vi "constants3.vi"() -> ()   [LabVIEW 2020]
panel:
  out "Robot_Width (in)":dbl
  out "Robot_Length (in)":dbl
  out "Angle_from_LL_to_Horizontal (deg)":dbl
  out "Height_from_LL_To_Ground_(in)":dbl
  out "Legal_Shooter_Setpoints":string[](array[string])
  out "Legal_Pipelines":string[](array[string])
  out "Legal_Actuator_Names":string[](array[string])
  out "Legal_Drivers":string[](array[string])
  out "Legal_Robots":string[](array[string])
  out "Legal_Auto_Plays":string[](array[string])
  out "Max_Robot_Ground_Speed_(ft/s)":dbl
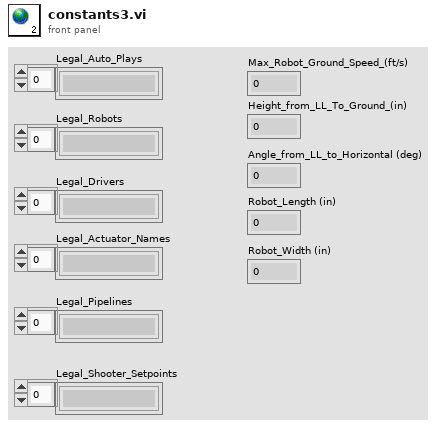
[diagram p1: front panel]
diagram:
